vi "Write Mode.vi"(8 "error in (no error)":errorcluster, 10 "Operational Mode":T1, 11 "Flip Mirror Containter in":refnum<class "Flip Mirror Containter.lvclass">) -> (0 "error out":errorcluster, 3 "Flip Mirror Containter out":refnum<class "Flip Mirror Containter.lvclass">)   [LabVIEW 2016, in "Flip Mirror Containter.lvclass"]
uses:
  Flip Mirror Containter.lvclass
  Controls/Operational Modes.ctl
  Flip Mirror Containter.lvclass/Flip Mirror Containter.ctl
  SolarMir.lvclass
  ThArMir.lvclass
  ExtFlatMir.lvclass
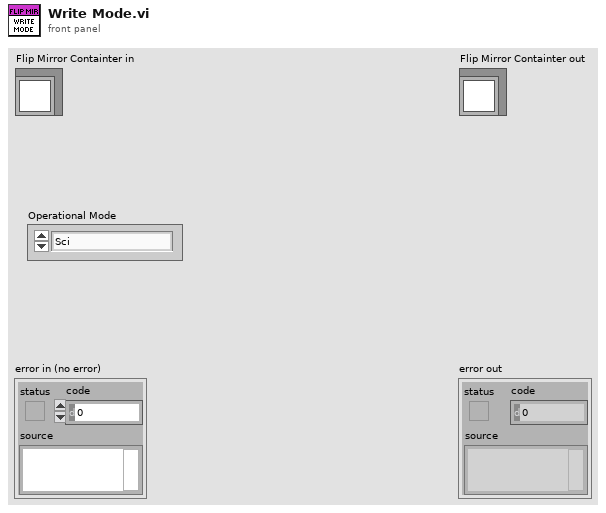
[diagram p1: front panel]
types:
  T1 = typedef "Operational Modes.ctl" = enum16{"Sci", "Sci-LFC", "Solar", "Solar-LFC", "LFC", "LFC-Sim", "LFC-Both", "ThAr", "ThAr-LFC", "Flat", "ExtFlat", "ExtFlat-Sim", "ExtFlat-Both", "Qtz", "ExtQtz", "ExtQtz-Sim", "ExtQtz-Both", "Dark", "Manual", "Off"}
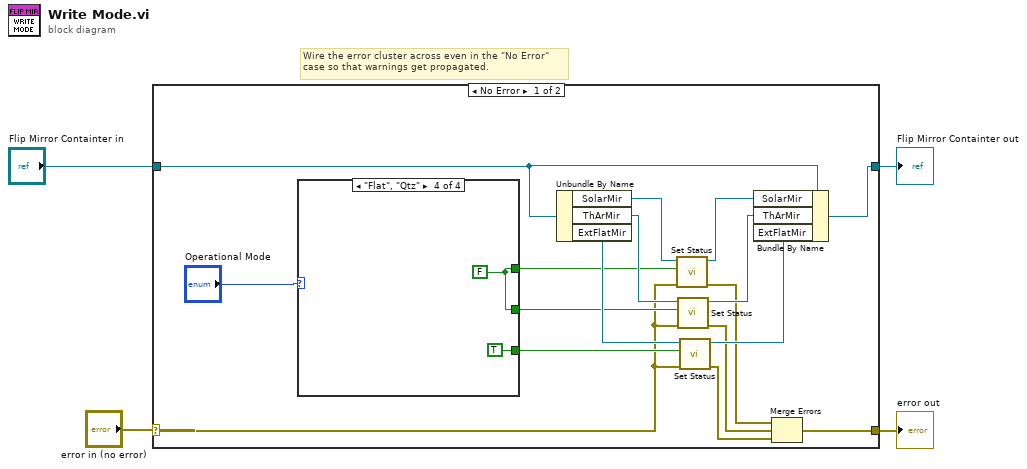
[diagram p0: block diagram]
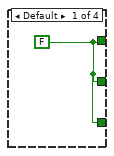
[diagram p2: hidden frame]
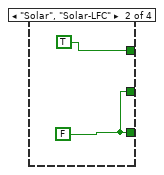
[diagram p3: hidden frame]
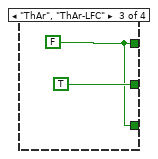
[diagram p4: hidden frame]
diagram:
  # "Wire the error cluster across even in the \"No Error\"\ncase so that warnings get propagated."
  n1 = case shown="No Error" "error in (no error)" {
    selector: "error in (no error)" -> [w9 w30]
    tunnel: [w8 w30] -> w3
    tunnel: [w19 w29] -> w1
    tunnel: "Flip Mirror Containter in" -> [w20 w29]
    frame No Error {
      n2 = case shown="\"Flat\", \"Qtz\"" "Operational Mode" {
        tunnel: [w22 TRUE w25 w27] -> w12
        tunnel: [w22 w23 TRUE w27] -> w11
        tunnel: [w22 w23 w25 TRUE] -> w10
        frame Default {
          w22 = FALSE
        }
        frame "Solar", "Solar-LFC" {
          w23 = FALSE
        }
        frame "ThAr", "ThAr-LFC" {
          w25 = FALSE
        }
        frame "Flat", "Qtz" {
          w27 = FALSE
        }
      }
      n3 = Unbundle By Name(w20) -> ("SolarMir"=w18:refnum<class "SolarMir.lvclass">, "ThArMir"=w16:refnum<class "ThArMir.lvclass">, "ExtFlatMir"=w15:refnum<class "ExtFlatMir.lvclass">)
      n4 = call-dynamic "Set Status.vi"("error in (no error)"=w9, "Status"=w12, "FlipMir in"=w18) -> ("error out"=w5:errorcluster, "FlipMir out"=w17:refnum<class "SolarMir.lvclass">)  [unwired: 7 in]
      n5 = call-dynamic "Set Status.vi"("error in (no error)"=w9, "Status"=w11, "FlipMir in"=w16) -> ("error out"=w6:errorcluster, "FlipMir out"=w14:refnum<class "ThArMir.lvclass">)  [unwired: 7 in]
      n6 = call-dynamic "Set Status.vi"("error in (no error)"=w9, "Status"=w10, "FlipMir in"=w15) -> ("error out"=w7:errorcluster, "FlipMir out"=w13:refnum<class "ExtFlatMir.lvclass">)  [unwired: 7 in]
      n7 = Bundle By Name(cluster=w20, "SolarMir"=w17, "ThArMir"=w14, "ExtFlatMir"=w13) -> (w19:refnum<class "Flip Mirror Containter.lvclass">)
      n8 = Merge Errors(w5, w6, w7) -> (w8:errorcluster)
    }
    frame Error {
    }
  }
  "error out" <- w3
  "Flip Mirror Containter out" <- w1
